vi "server2.vi"() -> ()   [LabVIEW 2018]
panel:
  out "concatenated string":string
  in  "Text.Scroll Position":u32
  out "current time":timestamp
  out "time string":string
  out "date string":string
  out "Boolean":bool
  out "data out 2":string
  out "data out":string
  out "error out":errorcluster
  in  "?":bool
  out "Chat":string
  in  "?":string
  out "bytes written":i32=5
  in  "?":bool
  in  "?":bool
  out "remote address":string="ulk412w7x64c04"
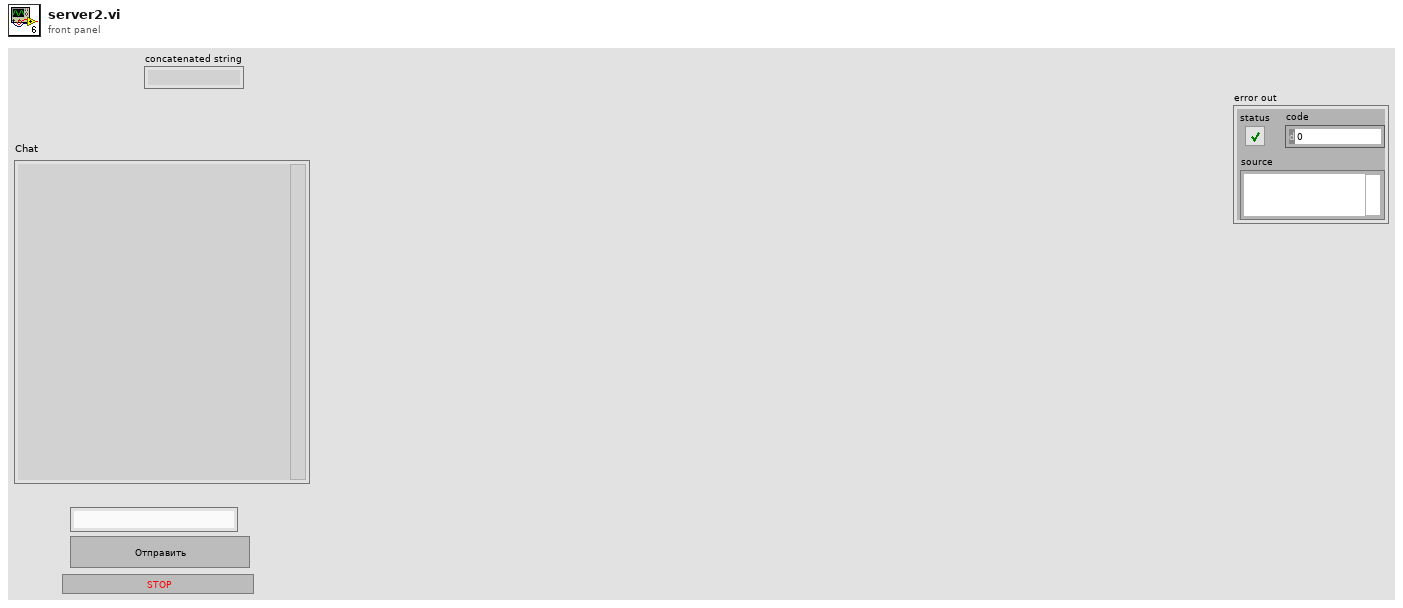
[diagram p1: front panel]
types:
  T1 = enum16{"Standard", "Buffered", "CRLF", "Immediate"}
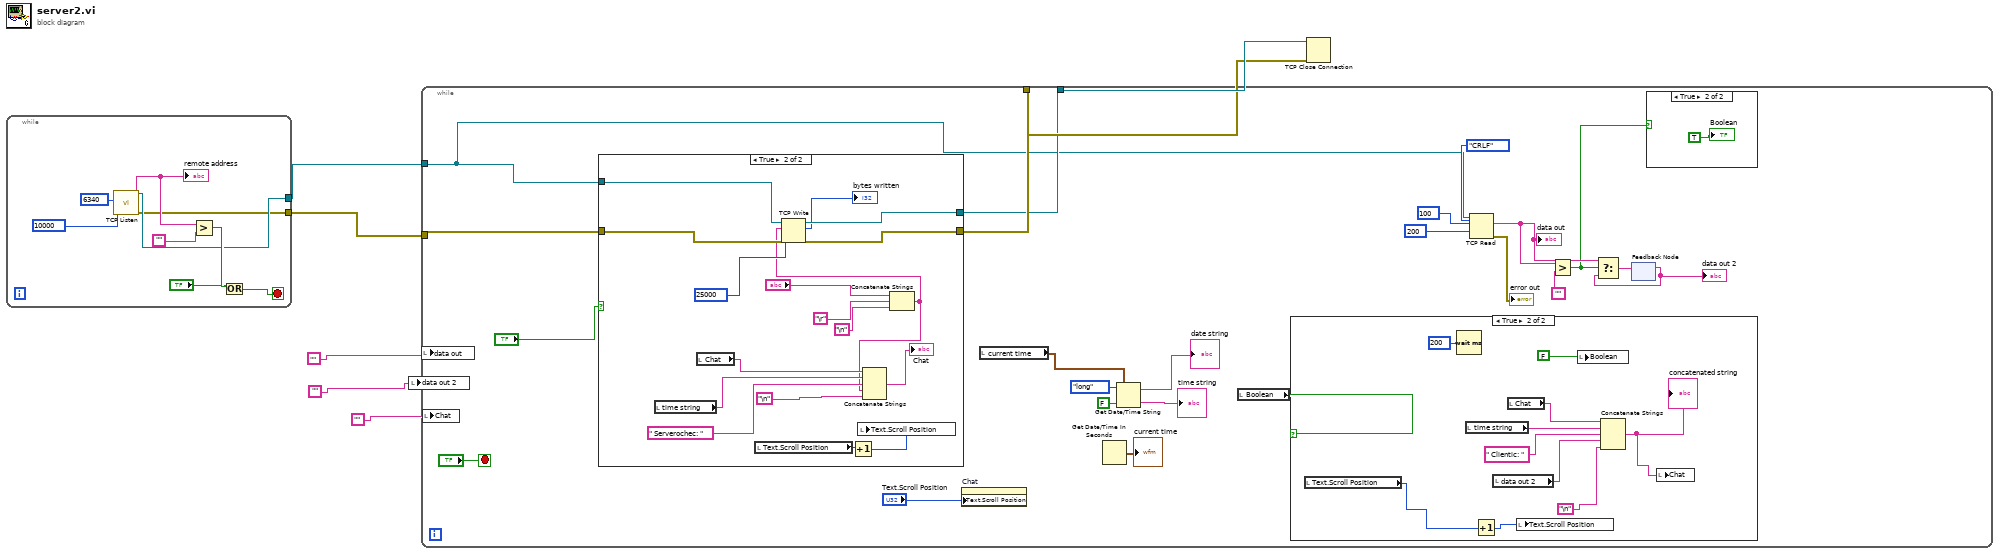
[diagram p0: block diagram]
diagram:
  n1 = while {
    tunnel: [w9] -> w7
    tunnel: [w8] -> w6
    stop <- w12 stop-if-true
    n2 = call <vilib>:"TCP Listen.vi"("timeout ms (wait forever: -1)"=10000, "port"=u16 6340) -> ("error out"=w8:errorcluster, "remote address"=w10:string, "connection ID"=w9:refnum<k5>)  [unwired: 5 in, 2 out]
    "remote address" <- w10
    n3 = Greater?(x=w10, y="") -> (0:w14:bool)
    n4 = Or(x=w14, y="?") -> (x .or. y?=w12:bool)
  }
  n5 = local write "data out 2"("") -> ()
  n6 = while {
    tunnel: w7 -> [w24]
    tunnel: w6 -> [w39]
    tunnel: [w25] -> w5
    tunnel: [w26] -> w4
    stop <- "?" stop-if-true
    n7 = case shown="True" "?" {
      tunnel: w24 -> [_ w64]
      tunnel: w39 -> [_ w63]
      tunnel: [_ w62] -> w25
      tunnel: [_ w61] -> w26
      frame False {
      }
      frame True {
        n8 = local read "time string"() -> (w57:string)
        n9 = local read "Chat"() -> (w58:string)
        n10 = local read "Text.Scroll Position"() -> (w52:u32)
        n11 = Increment(x=w52) -> (x+1=w51:u32)
        n12 = local write "Text.Scroll Position"(w51) -> ()
        n13 = Concatenate Strings("?", "\r", "\n") -> (w54:string)
        n14 = TCP Write(connection ID=w64, data in=w54, error in (no error)=w63, 9:25000 ("timeout ms (25000)")) -> (connection ID out=w62:refnum<k5>, bytes written=→"bytes written":i32, error out=w61:errorcluster)
        n15 = Concatenate Strings(w58, w57, " Serverochec: " ("string"), w54, "\n") -> (→"Chat":string)
      }
    }
    n16 = property on="Chat" class="Str"("Text.Scroll Position"="Text.Scroll Position") -> ()  [unwired: 2 in, 2 out]
    n17 = local read "current time"() -> (w18:timestamp)
    n18 = Get Date/Time In Seconds() -> (seconds since 1Jan1904=→"current time":timestamp)
    n19 = Get Date/Time String(date format (0)=enum16{"short", "long", "abbreviated"}."long", seconds (now)=w18, want seconds? (F)=FALSE) -> (date string=→"date string":string, time string=→"time string":string)
    n20 = local read "Boolean"() -> (w27:bool)
    n21 = case shown="True" w27 {
      frame False {
      }
      frame True {
        n22 = local read "Text.Scroll Position"() -> (w40:u32)
        n23 = Wait (ms)(milliseconds to wait=u32 200) -> ()  [unwired: 1 out]
        n24 = local read "time string"() -> (w45:string)
        n25 = Increment(x=w40) -> (x+1=w41:u32)
        n26 = local read "data out 2"() -> (w43:string)
        n27 = local read "Chat"() -> (w46:string)
        n28 = local write "Text.Scroll Position"(w41) -> ()
        n29 = local write "Boolean"(FALSE ("Boolean")) -> ()
        n30 = Concatenate Strings(w46, w45, " Clientic: " ("string"), w43, "\n") -> (w47:string)
        "concatenated string" <- w47
        n31 = local write "Chat"(w47) -> ()
      }
    }
    n32 = TCP Read(connection ID=w24, bytes to read=100, 7:T1."CRLF" ("mode (standard)"), 9:200 ("timeout ms (25000)")) -> (data out=w32:string, error out=→"error out":errorcluster)  [unwired: 1 in, 1 out]
    "data out" <- w32
    n33 = Greater?(x=w32, y="") -> (0:w28:bool)
    n34 = feedback #1() -> (w30:string)  [unwired: 1 in]
    "data out 2" <- w30
    n35 = Select(t=w32, s=w28, f=w30) -> (s? t:f=w31:string)
    n36 = feedback-in #1(w31) -> ()
    n37 = case shown="True" w28 {
      frame False {
      }
      frame True {
        "Boolean" <- TRUE ("Boolean")
      }
    }
  }
  n38 = local write "data out"("") -> ()
  n39 = local write "Chat"("") -> ()
  n40 = TCP Close Connection(connection ID=w5, error in (no error)=w4) -> ()  [unwired: 1 in, 2 out]
